vi "Write RP Transceiver.vi"(8 "error in (no error)":errorcluster, 10 "RP Transceiver.lvclass":refnum<class "RP Transceiver.lvclass">, 11 "Red Pitaya Transceiver Driver in":refnum<class "Red Pitaya Transceiver Driver.lvclass">) -> (0 "error out":errorcluster, 3 "Red Pitaya Transceiver Driver out":refnum<class "Red Pitaya Transceiver Driver.lvclass">)   [LabVIEW 2016, in "Red Pitaya Transceiver Driver.lvclass"]
uses:
  Red Pitaya Transceiver Driver.lvclass
  RP Transceiver/RP Transceiver.lvclass
  Red Pitaya Transceiver Driver.lvclass/Red Pitaya Transceiver Driver.ctl
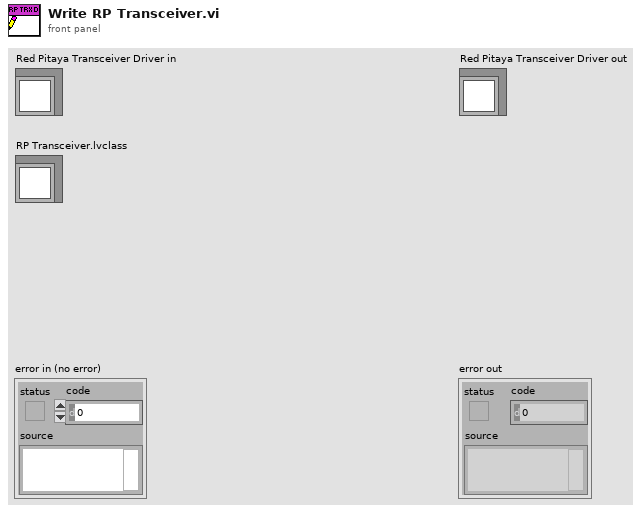
[diagram p1: front panel]
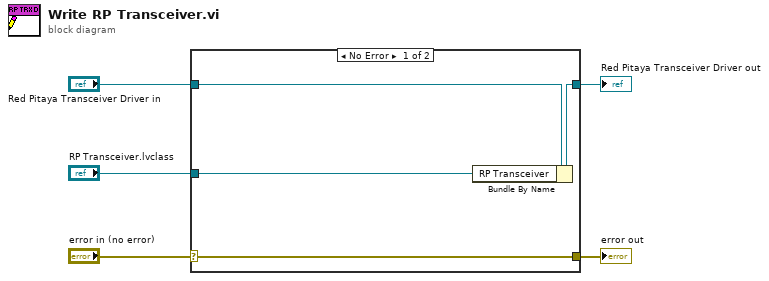
[diagram p0: block diagram]
diagram:
  n1 = case shown="No Error" "error in (no error)" {
    selector: "error in (no error)" -> [w9 w10]
    tunnel: [w9 w10] -> w4
    tunnel: [w7 w11] -> w2
    tunnel: "Red Pitaya Transceiver Driver in" -> [w8 w11]
    tunnel: "RP Transceiver.lvclass" -> [w6 _]
    frame No Error {
      n2 = Bundle By Name(cluster=w8, "RP Transceiver"=w6) -> (w7:refnum<class "Red Pitaya Transceiver Driver.lvclass">)
    }
    frame Error {
    }
  }
  "error out" <- w4
  "Red Pitaya Transceiver Driver out" <- w2
